vi "UHR-Fleezers Control (fpga) - 9.4.vi"() -> ()   [LabVIEW 2009]
doc: "UHR-Fleezers Instrument Control Code (fpga)"
uses:
  <vilib>/Platform/TimedLoop/XDataNode/XDataNode.xnode
  <vilib>/Platform/TimedLoop/XDataNode/loadlvalarms.vi
  <vilib>/Platform/TimedLoop/XDataNode/timing_clust.ctl
  <vilib>/Platform/TimedLoop/XDataNode/nitl_modes.ctl
  <vilib>/Platform/TimedLoop/XDataNode/wakeup.ctl
  <vilib>/eio/EIONode/EIONode.xnode
  <vilib>/rvi/eio/nirviEIOImplementation/nirviEIOImplementation.xnode
  <vilib>/rvi/eio/common/nirviEmuTemplateMethod_noerrors.vi
  <vilib>/rvi/eio/common/nirviEmuClasses.ctl
  <vilib>/eio/EIOMethodNode/EIOMethodNode.xnode
  <vilib>/rvi/eio/nirviEIOMethodImplementation/nirviEIOMethodImplementation.xnode
  <vilib>/rvi/DataTransferAndStorage/Container/XNode/niFpgaContainer.xnode
  <vilib>/rvi/interface/RandomDataEmulation/niFpgaRandomDataHandleErrors.vi
  <vilib>/rvi/interface/RandomDataEmulation/nirviRandomDataFPGAFIFO.vi
  <vilib>/rvi/DataTransferAndStorage/Container/Common/niFpgaContainerMethod.ctl
  <vilib>/rvi/DataTransferAndStorage/Container/Common/niFpgaTransferTypeControl.ctl
  <vilib>/Platform/TimedLoop/XDataNode/XDNodeRunTimeDep.lvlib
panel:
  in  "Tab Control":T1(tab)=enum."APD Counting"
  in  "AI Averages":u16=1 min=1 step=1
  in  "AI1 Sets to FIFO":T2={"Set 1"=TRUE, "Set 2"=TRUE, "Set 3"=FALSE}
  in  "N of AI1 Int Acq Sets":i16=2 min=1 max=3 step=1
  out "Number of AI channels":i16
  out "AI Late Counter":u32
  in  "ai count":u32=400
  out "AI late?":bool
  in  "+ phase":bool
  in  "Phase count adjustment":i16
  out "Relative phase":i16
  in  "DMA buffer timeout":i32
  in  "AI to FIFO":bool
  in  "Tab Control 2":T3(tab)
  in  "Swap F1 and F2":bool
  in  "Freq or Amp switch first":bool=TRUE
  in  "Cont. Scan":bool
  in  "Abort scan":bool
  in  "Cycles per step":u64
  in  "Scan BD":bool
  in  "Number of scans":u16
  in  "Scan steps":u64
  in  "Scan freq.  increment":i64
  out "Scanning":bool
  in  "Start scan":bool
  in  "OSK Bd 1":bool
  in  "Reset Bd 1":bool
  in  "RD":bool
  in  "PMODE":bool
  in  "OSK Bd 2":bool
  in  "Reset Bd 2":bool
  in  "Direct RF Box \nCommunication":bool
  in  "Data BD 2":u8 format="%08b"
  in  "Data BD 1":u8 format="%08b"
  in  "Address":u8 format="%02x"
  in  "Update Data":bool
  in  "FPGA Controls\n RF Box":bool
  in  "Number Interlace Cycles":u8=2 min=1 max=3
  in  "Interlace Off Parameters":u8=1 min=1 max=3
  in  "Interlace ON/OFF":bool
  out "DIO Relative phase":i16
  in  "Phase count adjustment (DIO)":i16
  in  "+ phase (DIO)":bool
  out "DIO Late Counter":u32
  out "DIO Late?":bool
  in  "DIO count 1 (ticks)":u32=400
  in  "DIO count 2 (ticks)":u32=400
  in  "DIO count 3 (ticks)":u32=400
  out "AI2 Y Sum Set 2":i16
  out "AI2 Y Sum Set 1":i16
  in  "FB Gains Set 1":T4={"proportional gain (Kc)"=10, "integral gain (Kc*Ts/Ti)"=5, "derivative gain (Kc*Td/Ts)"=0}
  in  "FB Setpoint Set 1":i16 min=0 step=1
  in  "FB Reset Set 1":bool
  in  "FB On/Off Set 1":bool
  in  "FB Reset Set 2":bool
  in  "FB On/Off Set 2":bool
  in  "FB Setpoint Set 2":i16 min=0 step=1
  in  "FB Gains Set 2":T4={"proportional gain (Kc)"=10, "integral gain (Kc*Ts/Ti)"=5, "derivative gain (Kc*Td/Ts)"=0}
  in  "FB output range 2":cluster{"output high":i16, "output low":i16}={"output high"=3000, "output low"=0}
  in  "FB output range 1":cluster{"output high":i16, "output low":i16}={"output high"=3000, "output low"=0}
  out "Scan I":u64
  in  "Amp switch delay":u16=5
  in  "Freq switch delay":u16
  in  "BD 2 Amplitude 1":u16
  in  "BD 1 Amplitude 1":u16
  in  "BD 2 Frequency 1":u64
  in  "BD 1 Frequency 1":u64
  in  "BD 2 Amplitude 2":u16
  in  "BD 1 Amplitude 2":u16
  in  "BD 2 Frequency 2":u64
  in  "BD 1 Frequency 2":u64
  in  "BD 2 Amplitude 3":u16
  in  "BD 1 Amplitude 3":u16
  in  "BD 2 Frequency 3":u64
  in  "BD 1 Frequency 3":u64
  out "Numeric":i32
  out "AO2 2":i16
  out "AO1 2":i16
  in  "1D or 2D Scan?":bool
  in  "Abort scan (MCL)":bool
  in  "MCL Scan Axis":bool
  in  "Cont. Scan (MCL)":bool
  out "Scan I (MCL)":u64
  in  "Number of scans (MCL)":u16
  out "Scanning MCL":bool
  in  "Scan steps (MCL)":u64
  in  "Cycles per step (MCL)":u64
  in  "Scan freq.  increment (MCL)":i16
  in  "Start scan (MCL)":bool
  in  "AO2":i16
  in  "AO1":i16
  out "MCL Late Counter":u32
  out "MCL Late?":bool
  in  "MCL count":u32=800
  out "MCL Relative Phase":i16
  in  "Phase count adjustment (MCL)":i16
  in  "+ phase (MCL)":bool
  in  "APD2 Trigger on Edge?":bool=TRUE
  in  "APD1 Trigger on Edge?":bool=TRUE
  in  "APD Gate Operating Mode":u8 max=2 step=1
  in  "Invert APD Gate":bool
  in  "APD Gate OFF Count":u32=100
  in  "APD Gate ON Count":u32=300
  out "APD 1 Gate Late Counter":u32
  out "APD 1 Gate Late?":bool
  out "APD 1 Gate Relative Phase":i16
  in  "Phase count adjustment (APD 1 Gate)":i16
  in  "+ phase (APD 1 Gate)":bool
  out "APD 2 Counts 0":u32
  out "APD 2 Counts 1":u32
  out "APD 1 Counts 0":u32
  out "APD 1 Counts 1":u32
  out "APD out state":bool
  in  "APD 2 AO offset":i16
  in  "APD 1 AO offset":i16
  in  "APD 2 AO scale factor":i16=1
  in  "APD 1 AO scale factor":i16=1
  in  "APD to FIFO":bool
  in  "APD Acq Rate Count":u32=20000000
  out "APD Acq Late Counter":u32
  out "APD Acq Late?":bool
  out "APD Acq Relative Phase":i16
  in  "Phase Count Adjustment (APD Acq)":i16
  in  "+ phase (APD Acq)":bool
  in  "Phase count adjustment (APD 2 Gate)":i16
  out "APD 2 Gate Late Counter":u32
  out "APD 2 Gate Late?":bool
  out "APD 2 Gate Relative Phase":i16
  in  "+ phase (APD 2 Gate)":bool
  in  "Green Filter Flipper":bool
  out "Green FB Signals":T5
  in  "Green FB Count":u32=1200
  out "Green Late Counter":u32
  out "Green FB Late?":bool
  out "Green FB Relative Phase":i16
  in  "Phase count adjustment (Green FB)":i16=10
  in  "+ phase (Green FB)":bool
  out "Green FB Sum":i16
  in  "Green int current ON count adj":u32=150
  in  "Current Out":u16=30000
  in  "Green FB On/Off":bool
  in  "Green FB Setpoint":i16=250 min=0 step=1
  in  "Green FB Gains":T4={"proportional gain (Kc)"=10, "integral gain (Kc*Ts/Ti)"=5, "derivative gain (Kc*Td/Ts)"=0}
  in  "Green FB Reset":bool
  in  "Operating Mode 2":u8=2 max=2 step=1
  in  "Invert GI 2":bool
  in  "Green interlace OFF count 2":u32=900
  in  "Green interlace ON count 2":u32=300
  out "GI Late Counter 2":u32
  out "GI Late? 2":bool
  out "GI Relative phase 2":i16
  in  "Phase count adjustment (GI) 2":i16=20
  in  "+ phase (GI) 2":bool
  in  "Green interlace OFF count":u32=100
  out "GI Relative phase":i16
  in  "Phase count adjustment (GI)":i16
  in  "+ phase (GI)":bool
  out "GI Late?":bool
  in  "Green interlace ON count":u32=300
  out "GI Late Counter":u32
  in  "Invert GI":bool
  in  "Operating Mode":u8 max=2 step=1
  in  "Connector0/DIO9":bool
  in  "Connector1/DIO32":bool
  in  "Connector1/DIO33":bool
  in  "Connector1/DIO34":bool
  in  "Chassis2/Mod4/AO1":u16
  in  "Extra DO Counts":u32=40000
  # "Only one of these can be on\nat a time:"
  # "Raster Scan AOD"
  # "1 (X)"
  # "2 (Y)"
  # "IR Intensity Feedback (RF BD 1)"
  # "AO1 (Y)"
  # "2D"
  # "1D"
  # "AO2 (X)"
  # "APD AO for aligning"
  # "Detection Loop"
  # "Green fluorescent laser digital gate interlacing loop"
  # "0 Forced ON\n1 Forced OFF\n2 Interlacing"
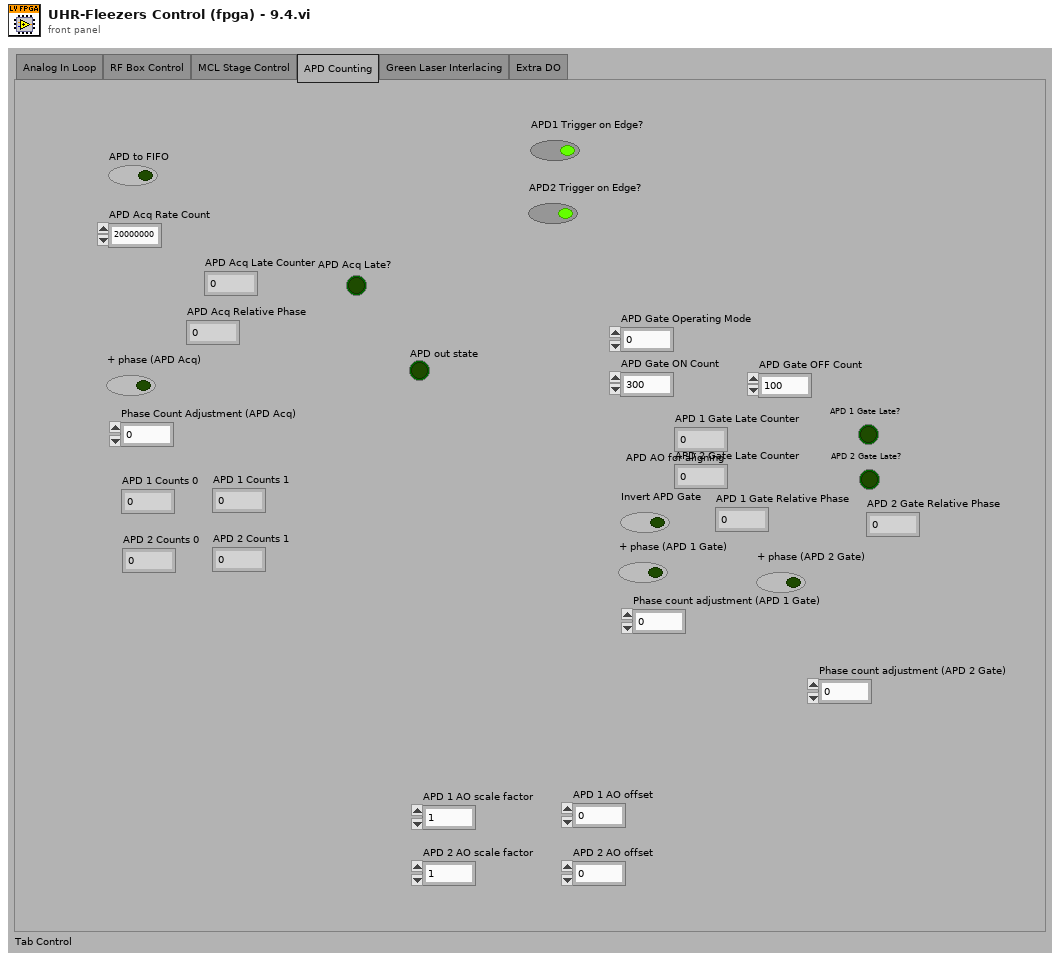
[diagram p1: front panel]
types:
  T1 = enum32{"Analog In Loop", "RF Box Control", "MCL Stage Control", "APD Counting", "Green Laser Interlacing", "Extra DO"}
  T2 = cluster{"Set 1":bool, "Set 2":bool, "Set 3":bool}
  T3 = enum32{"Controls", "Interlacing Frequency and Amplitude Values"}
  T4 = cluster{"proportional gain (Kc)":i16, "integral gain (Kc*Ts/Ti)":i16, "derivative gain (Kc*Td/Ts)":i16}
  T5 = cluster{"Green FB Ch 0":i16, "Green FB Ch 1":i16, "Green FB Ch 2":i16}
  T6 = typedef "nirviEmuClasses.ctl" = enum16{"IO Read", "IO Write", "Method", "Property Read", "Property Write"}
  T7 = typedef "XDNodeRunTimeDep.lvlib/timing_clust.ctl" = cluster{"Expected End [f-1]":u64, "Actual End [f-1]":u64, "Finished Late? [f-1]":bool, "Expected End [i-1]":u64, "Actual End [i-1]":u64, "Finished Late? [i-1]":bool, "Expected Start [i]":u64, "Actual Start [i]":u64, "Expected Start [f]":u64, "Actual Start [f]":u64, "Source Name":string, "Structure Name":string, "Period":i64, "Deadline":i64, "Offset":i64, "Start":i64, "Priority":i32, "Timeout":i32, "Mode":T8, "Wakeup Reason":T9, "Error":errorcluster, "Source Type":string, "Secondary Source Type":string, "Global End Time":u64, "Global Start Time":u64, "Frame Duration":u64, "Iteration Duration":u64, "Assigned CPU":i32, "I/O Scan Engine Mode":u32}
  T8 = typedef "XDNodeRunTimeDep.lvlib/nitl_modes.ctl" = enum32{"No Change", "Process missed periods, maintain original phase", "Discard missed periods, maintain original phase", "Process missed periods, ignore original phase", "Discard missed periods, ignore original phase"}
  T9 = typedef "XDNodeRunTimeDep.lvlib/wakeup.ctl" = enum32{"Normal", "Aborted", "Asynchronous wakeup", "Timing source error", "Timed loop error", "Timeout"}
  T10 = typedef "niFpgaContainerMethod.ctl" = enum16{"Write", "Read", "Clear", "Get Number of Elements to Write", "Get Number of Elements to Read", "Enable", "Disable", "Flush and Disable", "Get Stream State"}
  T11 = typedef "niFpgaTransferTypeControl.ctl" = enum16{"Target-Scoped", "Host to Target - DMA", "Target to Host - DMA", "Peer to Peer Reader", "Peer to Peer Writer", "Bidirectional"}
  T12 = cluster{"Chassis2/Mod1/AI0":i16, "Chassis2/Mod1/AI1":i16, "Chassis2/Mod1/AI2":i16}
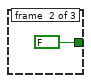
[diagram p2: hidden frame]
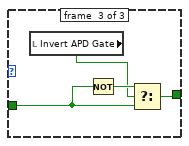
[diagram p3: hidden frame]
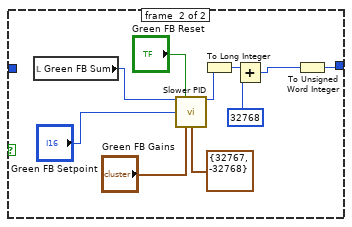
[diagram p4: hidden frame]
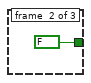
[diagram p5: hidden frame]
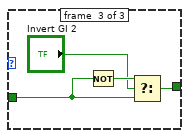
[diagram p6: hidden frame]
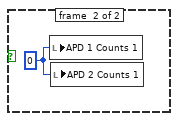
[diagram p7: hidden frame]
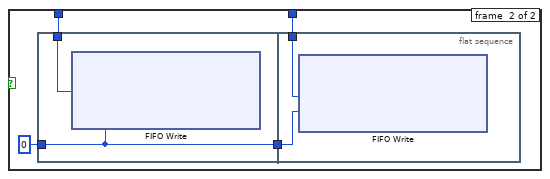
[diagram p8: hidden frame]
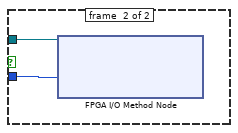
[diagram p9: hidden frame]
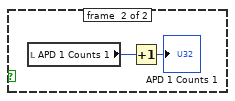
[diagram p10: hidden frame]
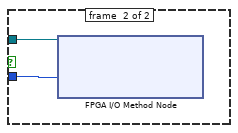
[diagram p11: hidden frame]
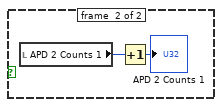
[diagram p12: hidden frame]
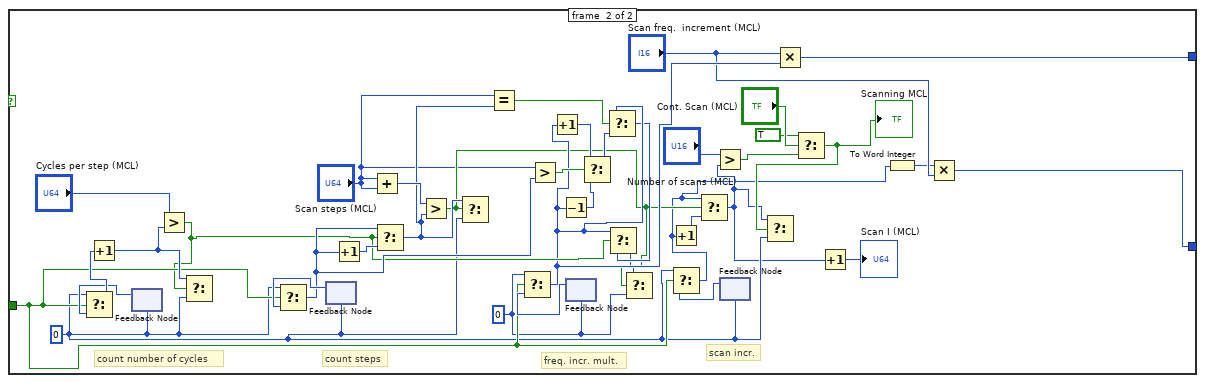
[diagram p13: hidden frame]
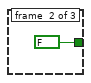
[diagram p14: hidden frame]
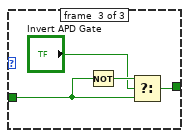
[diagram p15: hidden frame]
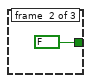
[diagram p16: hidden frame]
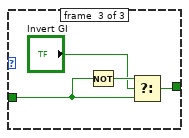
[diagram p17: hidden frame]
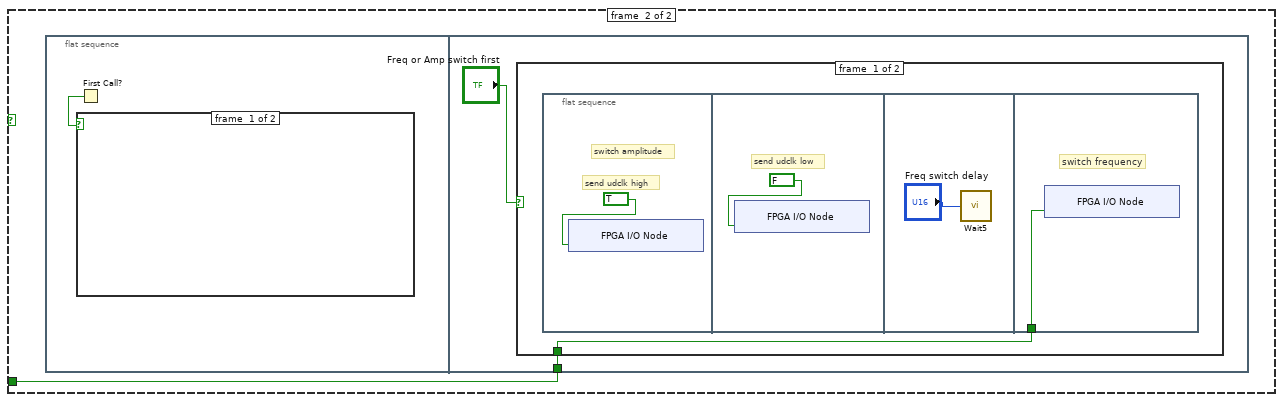
[diagram p18: hidden frame]
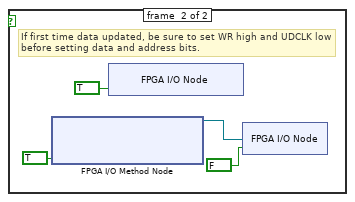
[diagram p19: hidden frame]
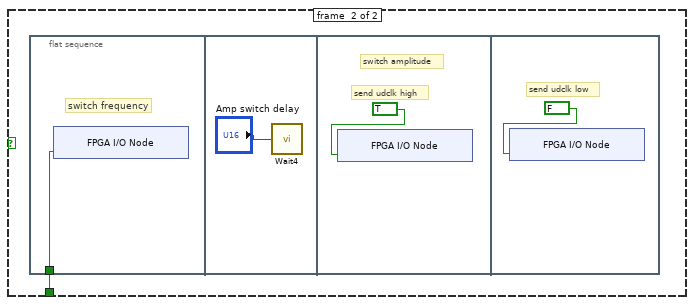
[diagram p20: hidden frame]
diagram:
  w2 = FALSE
  # "timing array current index"
  # "timing array"
  # "timing counter (phase adjusted here)"
  # "late counter"
  n1 = flat-sequence "FPGA initialization to do before running any of the loops" {
    tunnel: [u32 0 ("DIO count 3 (ticks)")] -> w1
    tunnel: [w10] -> _
    frame #0 {
      # "This is a kludge to let host programs know how many channels of data are in the DMA stream.  Set by hand."
      # "Start up expansion chassis early\nto avoid delays later"
      # "This pin controls udclk on the RF boards.\nWhen initially configuring the boards, this pin needs to be\nconfigured as a high impedance input.  Later it will be switched\nto an output."
      # "Initial setting of DIO data and \naddress to low (before reset).  \nThis needs to happen before the other\ncontrol method loops execute."
      n2 = xnode "FPGA I/O Node"("Chassis2/Mod4/AO0"=u16 0) -> ("Chassis2/Mod1/AI0"=w10:i16)  [unwired: 2 in, 2 out]
      n3 = xnode "FPGA I/O Method Node"("Enable"=FALSE) -> ()  [unwired: 1 in, 1 out]
      n4 = xnode "FPGA I/O Node"("Connector1/DIO0"=FALSE, "Connector1/DIO1"=FALSE, "Connector1/DIO2"=FALSE, "Connector1/DIO3"=FALSE, "Connector1/DIO4"=FALSE, "Connector1/DIO5"=FALSE, "Connector1/DIO6"=FALSE, "Connector1/DIO7"=FALSE, "Connector1/DIO8"=FALSE, "Connector1/DIO9"=FALSE, "Connector1/DIO10"=FALSE, "Connector1/DIO11"=FALSE, "Connector1/DIO12"=FALSE, "Connector1/DIO13"=FALSE, "Connector1/DIO15"=FALSE, "Connector1/DIO20"=FALSE, "Connector1/DIO21"=FALSE, "Connector1/DIO22"=FALSE, "Connector1/DIO23"=FALSE, "Connector1/DIO24"=FALSE, "Connector1/DIO25"=FALSE, "Connector1/DIO26"=FALSE, "Connector1/DIO27"=FALSE, "Connector1/DIO14"=FALSE) -> ()  [unwired: 24 in, 24 out]
      "Number of AI channels" <- i16 12 ("Number of AI channels")
    }
  }
  n5 = local read "AO1"() -> (w6:i16)
  n6 = local read "AO2"() -> (w5:i16)
  n7 = node-c288() -> (w4:T7)  [unwired: 1 in]
  n8 = while "APD 1 Counter" {
    tunnel: w1 -> [_]
    stop <- FALSE stop-if-true
    n9 = flat-sequence {
      frame #0 {
        n10 = case shown="False" "APD1 Trigger on Edge?" {
          tunnel: refnum<k21> "Connector0/DIO0" ("APD 1 DO") -> [w398 w423]
          tunnel: -1 ("Timeout") -> [w397 w422]
          frame #0 {
            n11 = xnode "FPGA I/O Method Node"("FPGA I/O In"=w398, "Timeout"=w397) -> ()  [unwired: 2 out]
          }
          frame #1 {
            n12 = xnode "FPGA I/O Method Node"("FPGA I/O In"=w423, "Timeout"=w422) -> ()  [unwired: 2 out]
          }
        }
      }
      frame #1 {
        n13 = local read "APD out state"() -> (w447:bool)
        n14 = case shown="False" w447 {
          frame #0 {
            n15 = local read "APD 1 Counts 0"() -> (w449:u32)
            n16 = Increment(x=w449) -> (x+1=→"APD 1 Counts 0":u32)
          }
          frame #1 {
            n17 = local read "APD 1 Counts 1"() -> (w451:u32)
            n18 = Increment(x=w451) -> (x+1=→"APD 1 Counts 1":u32)
          }
        }
      }
    }
  }
  n19 = while "APD 2 Counter" {
    tunnel: w1 -> [_]
    stop <- FALSE stop-if-true
    n20 = flat-sequence {
      frame #0 {
        n21 = case shown="False" "APD2 Trigger on Edge?" {
          tunnel: refnum<k21> "Connector0/DIO1" ("APD 2 DO") -> [w457 w482]
          tunnel: -1 ("Timeout") -> [w456 w481]
          frame #0 {
            n22 = xnode "FPGA I/O Method Node"("FPGA I/O In"=w457, "Timeout"=w456) -> ()  [unwired: 2 out]
          }
          frame #1 {
            n23 = xnode "FPGA I/O Method Node"("FPGA I/O In"=w482, "Timeout"=w481) -> ()  [unwired: 2 out]
          }
        }
      }
      frame #1 {
        n24 = local read "APD out state"() -> (w506:bool)
        n25 = case shown="False" w506 {
          frame #0 {
            n26 = local read "APD 2 Counts 0"() -> (w508:u32)
            n27 = Increment(x=w508) -> (x+1=→"APD 2 Counts 0":u32)
          }
          frame #1 {
            n28 = local read "APD 2 Counts 1"() -> (w510:u32)
            n29 = Increment(x=w510) -> (x+1=→"APD 2 Counts 1":u32)
          }
        }
      }
    }
  }
  n30 = while "APD 2 Gating" {
    shift-right: [w514] -> _
    shift-left: w1 -> [w519]
    shift-right: [w513] -> _
    shift-left: w2 -> [w511]
    stop <- FALSE stop-if-true
    n31 = flat-sequence {
      tunnel: w519 -> [w522]
      tunnel: [w523] -> w517
      tunnel: [w522] -> w515
      tunnel: [w521] -> w512
      tunnel: w511 -> [w521]
      tunnel: [w526] -> w518
      tunnel: w517 -> [w526]
      tunnel: [w525] -> w516
      tunnel: w515 -> [w525]
      tunnel: w512 -> [w524]
      tunnel: [w580] -> w514
      tunnel: w518 -> [w598]
      tunnel: w516 -> [w596]
      tunnel: [w585] -> w513
      frame #0 {
        n32 = call "Loop Timer8"("Count(Ticks)"=w522) -> ("Tick Count(Ticks)"=w523:u32)
      }
      frame #1 {
        # "(need 4 channels/APD)"
        n33 = xnode "FPGA I/O Node"("Connector0/DIO8"=w524, "Connector0/DIO9"=w524, "Connector0/DIO10"=w524, "Connector0/DIO11"=w524) -> ()  [unwired: 4 in, 4 out]
      }
      frame #2 {
        n34 = local read "APD Gate ON Count"() -> (w573:u32)
        n35 = local read "APD Gate OFF Count"() -> (w572:u32)
        n36 = feedback #1(TRUE) -> (w587:bool)
        n37 = feedback #2(w598) -> (w574:u32)
        n38 = Not(x=w587) -> (.not. x?=w584:bool)
        n39 = Subtract(x=w598, y=w574) -> (x-y=w597:u32)
        n40 = Select(t=w573, s=w584, f=w572) -> (s? t:f=w589:u32)
        n41 = Subtract(x=w597, y=w596) -> (x-y=w590:u32)
        n42 = Subtract(x=w589, y=w590) -> (x-y=w579:u32)
        n43 = Greater?(x=w590, y=u32 0) -> (0:w592:bool)
        "APD 2 Gate Late?" <- w592
        n44 = Boolean To (0,1)(Boolean="+ phase (APD 2 Gate)") -> (0, 1=w577:i16)
        n45 = Multiply(x=w577, y="Phase count adjustment (APD 2 Gate)") -> (x*y=w575:i16)
        n46 = feedback #3(u32 0) -> (w594:u32)
        n47 = Increment(x=w594) -> (x+1=w593:u32)
        n48 = Select(t=w593, s=w592, f=w594) -> (s? t:f=w591:u32)
        "APD 2 Gate Late Counter" <- w591
        n49 = Add(x=w579, y=w575) -> (x+y=w580:u32)
        n50 = feedback #4(i16 0) -> (w582:i16)
        n51 = Subtract(x=w582, y=w575) -> (x-y=w581:i16)
        "APD 2 Gate Relative Phase" <- w581
        n52 = local read "APD Gate Operating Mode"() -> (w571:u8)
        n53 = case shown="2" w571 {
          tunnel: [TRUE FALSE w604] -> w585
          tunnel: w587 -> [_ _ w602]
          frame #0 {
          }
          frame #1 {
          }
          frame #2 {
            n54 = local read "Invert APD Gate"() -> (w601:bool)
            n55 = Not(x=w602) -> (.not. x?=w603:bool)
            n56 = Select(t=w603, s=w601, f=w602) -> (s? t:f=w604:bool)
          }
        }
      }
    }
  }
  n57 = while "DAQ AI set 1" {
    shift-right: [w605] -> _
    shift-left: w1 -> [w610]
    stop <- FALSE stop-if-true
    n58 = flat-sequence {
      tunnel: w610 -> [w620]
      tunnel: [w621] -> w608
      tunnel: [w620] -> w607
      tunnel: [w631] -> w618
      tunnel: [w630] -> w617
      tunnel: [w629] -> w616
      tunnel: [w628] -> w615
      tunnel: [w627] -> w614
      tunnel: [w626] -> w613
      tunnel: [w625] -> w612
      tunnel: [w624] -> w611
      tunnel: [w623] -> w609
      tunnel: w608 -> [w623]
      tunnel: w607 -> [w622]
      tunnel: [w622] -> w606
      tunnel: [w808] -> w605
      tunnel: w618 -> [w846]
      tunnel: w617 -> [w845]
      tunnel: w616 -> [w829]
      tunnel: w615 -> [w844]
      tunnel: w614 -> [w833]
      tunnel: w613 -> [w832]
      tunnel: w612 -> [w831]
      tunnel: w611 -> [w830]
      tunnel: w609 -> [w825]
      tunnel: w606 -> [w822]
      frame #0 {
        n59 = call "Loop Timer3"("Count(Ticks)"=w620) -> ("Tick Count(Ticks)"=w621:u32)
      }
      frame #1 {
        n60 = xnode "FPGA I/O Node"("Connector1/DIO31"=TRUE ("Connector1/DIO33")) -> ("Connector0/AI0"=w631:i16, "Connector0/AI1"=w630:i16, "Connector0/AI2"=w629:i16, "Connector0/AI3"=w628:i16, "Connector0/AI4"=w627:i16, "Connector0/AI5"=w626:i16, "Connector0/AI6"=w625:i16, "Connector0/AI7"=w624:i16)  [unwired: 9 in, 9 out]
      }
      frame #2 {
        # "Adjust phase after data acquired if button pressed"
        n61 = feedback #5(i16 1) -> (w837:i16)
        n62 = Increment(x=w837) -> (x+1=w843:i16)
        n63 = Greater?(x=w843, y="N of AI1 Int Acq Sets") -> (0:w840:bool)
        n64 = Select(t=i16 1, s=w840, f=w843) -> (s? t:f=w842:i16)
        n65 = feedback #6(FALSE ("AI to FIFO")) -> (w827:bool)
        n66 = case shown="1, Default" w837 {
          tunnel: w829 -> [w849 w853 _]
          tunnel: "AI1 Sets to FIFO" -> [w851 w855 w858]
          tunnel: [w850 w854 w857] -> w834
          tunnel: ["AI to FIFO" w852 w856] -> w826
          tunnel: w827 -> [_ w852 w856]
          frame #0 {
            n67 = Unbundle By Name(w851) -> ("Set 1"=w850:bool)
            "AI2 Y Sum Set 1" <- w849
          }
          frame #1 {
            n68 = Unbundle By Name(w855) -> ("Set 2"=w854:bool)
            "AI2 Y Sum Set 2" <- w853
          }
          frame #2 {
            n69 = Unbundle By Name(w858) -> ("Set 3"=w857:bool)
          }
        }
        n70 = And(x=w834, y=w826) -> (x .and. y?=w836:bool)
        n71 = case shown="True" w836 {
          tunnel: w846 -> [_ w863]
          tunnel: w845 -> [_ w864]
          tunnel: w829 -> [_ w865]
          tunnel: w844 -> [_ w866]
          tunnel: w833 -> [_ w870]
          tunnel: w832 -> [_ w869]
          tunnel: w831 -> [_ w868]
          tunnel: w830 -> [_ w867]
          frame #0 {
          }
          frame #1 {
            n72 = Greater?(x="AI Averages", y=u16 1) -> (0:w861:bool)
            n73 = case shown="True" w861 {
              tunnel: w870 -> [w881 w938]
              tunnel: w869 -> [w880 w937]
              tunnel: w868 -> [w879 w936]
              tunnel: w867 -> [w878 w935]
              tunnel: w866 -> [w877 w934]
              tunnel: w865 -> [w882 w933]
              tunnel: w864 -> [w883 w932]
              tunnel: w863 -> [w884 w931]
              tunnel: "AI Averages" -> [_ w918]
              tunnel: "DMA buffer timeout" -> [w872 w915]
              frame #0 {
                n74 = Join Numbers(hi=w884, lo=w883) -> ((hi.lo)=w876:u32)
                n75 = Join Numbers(hi=w882, lo=w877) -> ((hi.lo)=w875:u32)
                n76 = Join Numbers(hi=w881, lo=w880) -> ((hi.lo)=w874:u32)
                n77 = Join Numbers(hi=w879, lo=w878) -> ((hi.lo)=w873:u32)
                n78 = Build Array(w876, w875, w874, w873) -> (w871:u32[])
                n79 = for {
                  tunnel: w871 -> [w886] mode=indexing
                  tunnel: w872 -> [w887]
                  n80 = To Unsigned Long Integer(number=w886) -> (unsigned 32bit integer=w885:u32)
                  n81 = xnode ("FIFO Write")("Element"=w885, "Timeout"=w887) -> ()  [unwired: 1 in, 2 out]
                }
              }
              frame #1 {
                w922 = u16 0
                n82 = To Long Integer(number=w931) -> (32bit integer=w924:i32)
                n83 = To Long Integer(number=w932) -> (32bit integer=w941:i32)
                n84 = To Long Integer(number=w933) -> (32bit integer=w940:i32)
                n85 = To Long Integer(number=w934) -> (32bit integer=w939:i32)
                n86 = To Long Integer(number=w938) -> (32bit integer=w930:i32)
                n87 = To Long Integer(number=w937) -> (32bit integer=w929:i32)
                n88 = To Long Integer(number=w936) -> (32bit integer=w928:i32)
                n89 = To Long Integer(number=w935) -> (32bit integer=w927:i32)
                n90 = Build Array(w924, w941, w940, w939, w930, w929, w928, w927) -> (w913:i32[])
                n91 = feedback #7(w913) -> (w926:i32[])
                n92 = Add(x=w913, y=w926) -> (x+y=w925:i32[])
                n93 = feedback #8(w922) -> (w920:u16)
                n94 = Increment(x=w920) -> (x+1=w917:u16)
                n95 = Equal?(x=w917, y=u16 1) -> (x = y?=w916:bool)
                n96 = Select(t=w913, s=w916, f=w925) -> (s? t:f=w914:i32[])
                n97 = Greater Or Equal?(x=w917, y=w918) -> (x >= y?=w919:bool)
                n98 = Select(t=w922, s=w919, f=w917) -> (s? t:f=w921:u16)
                n99 = case shown="True" w919 {
                  tunnel: w914 -> [_ w943]
                  tunnel: w915 -> [_ w942]
                  frame #0 {
                  }
                  frame #1 {
                    n100 = for {
                      tunnel: w943 -> [w945] mode=indexing
                      tunnel: w942 -> [w946]
                      n101 = To Unsigned Long Integer(number=w945) -> (unsigned 32bit integer=w944:u32)
                      n102 = xnode ("FIFO Write")("Element"=w944, "Timeout"=w946) -> ()  [unwired: 1 in, 2 out]
                    }
                  }
                }
              }
            }
          }
        }
        n103 = feedback #9(w825) -> (w824:u32)
        n104 = Subtract(x=w825, y=w824) -> (x-y=w823:u32)
        n105 = Subtract(x=w823, y=w822) -> (x-y=w819:u32)
        n106 = Subtract(x="ai count", y=w819) -> (x-y=w809:u32)
        n107 = Greater?(x=w819, y=u32 0) -> (0:w817:bool)
        "AI late?" <- w817
        n108 = feedback #10(u32 0) -> (w815:u32)
        n109 = Increment(x=w815) -> (x+1=w814:u32)
        n110 = Select(t=w814, s=w817, f=w815) -> (s? t:f=w816:u32)
        "AI Late Counter" <- w816
        n111 = xnode "I/O Node"("Connector1/DIO31"=FALSE ("Connector1/DIO34")) -> ()  [unwired: 1 in, 1 out]
        n112 = Boolean To (0,1)(Boolean="+ phase") -> (0, 1=w811:i16)
        n113 = Multiply(x=w811, y="Phase count adjustment") -> (x*y=w805:i16)
        n114 = feedback #11(i16 0) -> (w807:i16)
        n115 = Add(x=w809, y=w805) -> (x+y=w808:u32)
        n116 = Subtract(x=w807, y=w805) -> (x-y=w806:i16)
        "Relative phase" <- w806
      }
    }
  }
  n117 = while "RF box board DIO control: parallel communication" {
    shift-right: [w991] -> _
    shift-left: w1 -> [w990]
    shift-right: [w989] -> _
    shift-left: FALSE ("Swap F1 and F2") -> [w988]
    stop <- FALSE stop-if-true
    n118 = flat-sequence {
      tunnel: w988 -> [w995]
      tunnel: w990 -> [w993]
      tunnel: [w995] -> w987
      tunnel: [w994] -> w986
      tunnel: [w993] -> w985
      tunnel: [w1001] -> w991
      tunnel: [w1000] -> w989
      tunnel: w987 -> [w999]
      tunnel: w986 -> [w997]
      tunnel: w985 -> [w996]
      frame #0 {
        n119 = call "Loop Timer"("Count(Ticks)"=w993) -> ("Tick Count(Ticks)"=w994:u32)
      }
      frame #1 {
        n120 = flat-sequence {
          tunnel: ["FPGA Controls\n RF Box"] -> w998
          tunnel: w999 -> [w1002]
          tunnel: [w1151] -> w1001
          tunnel: [w1171] -> w1000
          tunnel: w998 -> [w1170]
          tunnel: w997 -> [w1164]
          tunnel: w996 -> [w1161]
          frame #0 {
            n121 = case shown="True" "FPGA Controls\n RF Box" {
              tunnel: w1002 -> [_ w1004]
              frame #0 {
              }
              frame #1 {
                n122 = flat-sequence {
                  tunnel: w1004 -> [w1049]
                  frame #0 {
                    n123 = First Call?() -> (First Call?: T/F=w1005:bool)
                    n124 = case shown="True" w1005 {
                      frame #0 {
                      }
                      frame #1 {
                        # "If first time data updated, be sure to set WR high and UDCLK low\nbefore setting data and address bits."
                        n125 = xnode "FPGA I/O Method Node"("Enable"=TRUE) -> ("FPGA I/O Out"=w1007:refnum<k21>)  [unwired: 1 in]
                        n126 = xnode "FPGA I/O Node"("Connector1/DIO15"=TRUE) -> ()  [unwired: 1 in, 1 out]
                        n127 = xnode "FPGA I/O Node"("I/O Item"=FALSE ("Connector1/DIO30"), "FPGA I/O In"=w1007) -> ()  [unwired: 1 out]
                      }
                    }
                  }
                  frame #1 {
                    n128 = case shown="True" "Freq or Amp switch first" {
                      tunnel: w1049 -> [w1051 w1095]
                      frame #0 {
                        n129 = flat-sequence {
                          tunnel: w1051 -> [w1081]
                          frame #0 {
                            # "switch amplitude"
                            # "send udclk high"
                            n130 = xnode "FPGA I/O Node"("Connector1/DIO30"=TRUE ("Connector1/DIO15")) -> ()  [unwired: 1 in, 1 out]
                          }
                          frame #1 {
                            # "send udclk low"
                            n131 = xnode "FPGA I/O Node"("Connector1/DIO30"=FALSE ("Connector1/DIO15")) -> ()  [unwired: 1 in, 1 out]
                          }
                          frame #2 {
                            n132 = call "Wait5"("Count(Ticks)"="Freq switch delay") -> ()  [unwired: 1 out]
                          }
                          frame #3 {
                            # "switch frequency"
                            n133 = xnode "FPGA I/O Node"("Connector1/DIO36"=w1081) -> ()  [unwired: 1 in, 1 out]
                          }
                        }
                      }
                      frame #1 {
                        n134 = flat-sequence {
                          tunnel: w1095 -> [w1096]
                          frame #0 {
                            # "switch frequency"
                            n135 = xnode "FPGA I/O Node"("Connector1/DIO36"=w1096) -> ()  [unwired: 1 in, 1 out]
                          }
                          frame #1 {
                            n136 = call "Wait4"("Count(Ticks)"="Amp switch delay") -> ()  [unwired: 1 out]
                          }
                          frame #2 {
                            # "switch amplitude"
                            # "send udclk high"
                            n137 = xnode "FPGA I/O Node"("Connector1/DIO30"=TRUE ("Connector1/DIO15")) -> ()  [unwired: 1 in, 1 out]
                          }
                          frame #3 {
                            # "send udclk low"
                            n138 = xnode "FPGA I/O Node"("Connector1/DIO30"=FALSE ("Connector1/DIO15")) -> ()  [unwired: 1 in, 1 out]
                          }
                        }
                      }
                    }
                  }
                }
              }
            }
          }
          frame #1 {
            # "This is the prior cycle's on time"
            # "increment timing\nindex, reset to 0 if \nend of matrix"
            # "Reset to begginning (1) when number of cycles reached."
            # "timing index"
            # "build byte stacks for writing data\n(must correspond to addresses array constant)"
            # "Timing housekeeping"
            # "Adjust phase if late\n(maintains constant phase relationship between cycles)"
            n139 = feedback #12(u8 0 ("t")) -> (w1167:u8)
            n140 = Increment(x=w1167) -> (x+1=w1211:u8)
            n141 = Increment(x="Number Interlace Cycles") -> (x+1=w1206:u8)
            n142 = Equal?(x=w1211, y=w1206) -> (x = y?=w1213:bool)
            n143 = Select(t=u8 1, s=w1213, f=w1211) -> (s? t:f=w1166:u8)
            n144 = Increment(x=w1166) -> (x+1=w1208:u8)
            n145 = Equal?(x=w1208, y=w1206) -> (x = y?=w1209:bool)
            n146 = Select(t=u8 1, s=w1209, f=w1208) -> (s? t:f=w1205:u8)
            n147 = Select(t=w1205, s="Interlace ON/OFF", f="Interlace Off Parameters") -> (s? t:f=w1189:u8)
            n148 = case shown="1, Default" w1189 {
              tunnel: [w1285 "BD 1 Frequency 2" "BD 1 Frequency 3"] -> w1201
              tunnel: [w1284 "BD 2 Frequency 2" "BD 2 Frequency 3"] -> w1190
              tunnel: ["BD 2 Amplitude 1" "BD 2 Amplitude 2" "BD 2 Amplitude 3"] -> w1139
              tunnel: [w1273 w1343 "BD 1 Amplitude 3"] -> w1142
              frame #0 {
                w1280 = u8 0 ("f")
                n149 = local read "Scanning"() -> (w1286:bool)
                n150 = Or(x=w1286, y="Start scan") -> (x .or. y?=w1278:bool)
                n151 = Not(x="Abort scan") -> (.not. x?=w1276:bool)
                n152 = And(x=w1276, y=w1278) -> (x .and. y?=w1275:bool)
                n153 = case "Raster scan" shown="True" w1275 {
                  tunnel: [i16 0 w1332] -> w1281
                  tunnel: "Start scan" -> [_ w1317]
                  frame #0 {
                    n154 = local write "Scanning"(FALSE ("scanning")) -> ()
                  }
                  frame #1 {
                    w1301 = i64 0
                    w1300 = u64 0
                    # "scan incr."
                    # "freq. incr. mult."
                    # "count steps"
                    # "count number of cycles"
                    n155 = feedback #13(w1300) -> (w1329:u64)
                    n156 = Select(t=w1300, s=w1317, f=w1329) -> (s? t:f=w1331:u64)
                    n157 = Increment(x=w1331) -> (x+1=w1328:u64)
                    n158 = Greater?(x="Cycles per step", y=w1328) -> (0:w1310:bool)
                    n159 = Select(t=w1328, s=w1310, f=w1300) -> (s? t:f=w1327:u64)
                    n160 = feedback #14(w1300) -> (w1326:u64)
                    n161 = Select(t=w1300, s=w1317, f=w1326) -> (s? t:f=w1321:u64)
                    n162 = Increment(x=w1321) -> (x+1=w1325:u64)
                    n163 = Add(x="Scan steps", y="Scan steps") -> (x+y=w1324:u64)
                    n164 = Select(t=w1321, s=w1310, f=w1325) -> (s? t:f=w1305:u64)
                    n165 = Greater?(x=w1324, y=w1305) -> (0:w1304:bool)
                    n166 = Select(t=w1305, s=w1304, f=w1300) -> (s? t:f=w1322:u64)
                    n167 = Equal?(x="Scan steps", y=w1305) -> (x = y?=w1309:bool)
                    n168 = Greater?(x="Scan steps", y=w1321) -> (0:w1320:bool)
                    n169 = feedback #15(w1301) -> (w1323:i64)
                    n170 = Select(t=w1301, s=w1317, f=w1323) -> (s? t:f=w1307:i64)
                    n171 = Increment(x=w1307) -> (x+1=w1319:i64)
                    n172 = Decrement(x=w1307) -> (x-1=w1318:i64)
                    n173 = Select(t=w1319, s=w1320, f=w1318) -> (s? t:f=w1308:i64)
                    n174 = Select(t=w1307, s=w1309, f=w1308) -> (s? t:f=w1306:i64)
                    n175 = Select(t=w1307, s=w1310, f=w1306) -> (s? t:f=w1302:i64)
                    n176 = Select(t=w1302, s=w1304, f=w1301) -> (s? t:f=w1303:i64)
                    n177 = feedback #16(w1300) -> (w1316:u64)
                    n178 = Select(t=w1300, s=w1317, f=w1316) -> (s? t:f=w1312:u64)
                    n179 = Increment(x=w1312) -> (x+1=w1313:u64)
                    n180 = Select(t=w1312, s=w1304, f=w1313) -> (s? t:f=w1311:u64)
                    n181 = Greater?(x="Number of scans", y=w1311) -> (0:w1297:bool)
                    n182 = Multiply(x="Scan freq.  increment", y=w1307) -> (x*y=w1332:i64)
                    n183 = Select(t=TRUE, s="Cont. Scan", f=w1297) -> (s? t:f=w1296:bool)
                    "Scanning" <- w1296
                    n184 = Select(t=w1311, s=w1296, f=w1300) -> (s? t:f=w1314:u64)
                    n185 = Increment(x=w1311) -> (x+1=→"Scan I":u64)
                  }
                }
                n186 = case shown="True" "FB On/Off Set 1" {
                  tunnel: "BD 1 Amplitude 1" -> [w1334 _]
                  tunnel: [w1334 w1335] -> w1273
                  frame #0 {
                  }
                  frame #1 {
                    n187 = local read "AI2 Y Sum Set 1"() -> (w1337:i16)
                    n188 = call "Slower PID.vi"("process variable"=w1337, "reset?"="FB Reset Set 1", "setpoint"="FB Setpoint Set 1", "PID gains (x 2^8)"="FB Gains Set 1", "output range"="FB output range 1") -> ("output"=w1340:i16)  [unwired: 10 out]
                    n189 = To Unsigned Word Integer(number=w1340) -> (unsigned 16bit integer=w1335:u16)
                  }
                }
                n190 = Select(t=w1280, s="Scan BD", f=w1281) -> (s? t:f=w1279:i64)
                n191 = Select(t=w1281, s="Scan BD", f=w1280) -> (s? t:f=w1282:i64)
                n192 = Add(x=w1279, y="BD 2 Frequency 1") -> (x+y=w1284:u64)
                n193 = Add(x="BD 1 Frequency 1", y=w1282) -> (x+y=w1285:u64)
              }
              frame #1 {
                n194 = case shown="True" "FB On/Off Set 2" {
                  tunnel: [w1348 w1349] -> w1343
                  tunnel: "BD 1 Amplitude 2" -> [w1348 _]
                  frame #0 {
                  }
                  frame #1 {
                    n195 = local read "AI2 Y Sum Set 2"() -> (w1354:i16)
                    n196 = call "Slower PID.vi"("process variable"=w1354, "reset?"="FB Reset Set 2", "setpoint"="FB Setpoint Set 2", "PID gains (x 2^8)"="FB Gains Set 2", "output range"="FB output range 2") -> ("output"=w1351:i16)  [unwired: 10 out]
                    n197 = To Unsigned Word Integer(number=w1351) -> (unsigned 16bit integer=w1349:u16)
                  }
                }
              }
              frame #2 {
              }
            }
            n198 = feedback #17(w1164) -> (w1163:u32)
            n199 = Subtract(x=w1164, y=w1163) -> (x-y=w1162:u32)
            n200 = Select(t=w1166, s="Interlace ON/OFF", f="Interlace Off Parameters") -> (s? t:f=w1204:u8)
            n201 = Subtract "The error"(x=w1162, y=w1161) -> (x-y=w1159:u32)
            n202 = case shown="3" w1204 {
              tunnel: ["DIO count 1 (ticks)" "DIO count 2 (ticks)" "DIO count 3 (ticks)"] -> w1160
              frame #0 {
              }
              frame #1 {
              }
              frame #2 {
              }
            }
            n203 = Greater?(x=w1159, y=u32 0) -> (0:w1154:bool)
            "DIO Late?" <- w1154
            n204 = feedback #18(u32 0) -> (w1156:u32)
            n205 = Increment(x=w1156) -> (x+1=w1155:u32)
            n206 = Select(t=w1155, s=w1154, f=w1156) -> (s? t:f=w1157:u32)
            "DIO Late Counter" <- w1157
            n207 = Subtract(x=w1160, y=w1159) -> (x-y=w1152:u32)
            n208 = Boolean To (0,1)(Boolean="+ phase (DIO)") -> (0, 1=w1149:i16)
            n209 = Multiply(x=w1149, y="Phase count adjustment (DIO)") -> (x*y=w1145:i16)
            n210 = feedback #19(i16 0) -> (w1147:i16)
            n211 = Subtract(x=w1147, y=w1145) -> (x-y=w1146:i16)
            "DIO Relative phase" <- w1146
            n212 = Split Number(x=w1190) -> (hi(x)=w1195:u32, lo(x)=w1194:u32)
            n213 = Split Number(x=w1201) -> (hi(x)=w1200:u32, lo(x)=w1199:u32)
            n214 = Split Number(x=w1195) -> (lo(x)=w1193:u16)  [unwired: 1 out]
            n215 = Split Number(x=w1194) -> (hi(x)=w1192:u16, lo(x)=w1191:u16)
            n216 = Split Number(x=w1200) -> (lo(x)=w1198:u16)  [unwired: 1 out]
            n217 = Split Number(x=w1199) -> (hi(x)=w1197:u16, lo(x)=w1196:u16)
            n218 = Split Number(x=w1142) -> (hi(x)=w1144:u8, lo(x)=w1143:u8)
            n219 = Split Number(x=w1193) -> (hi(x)=w1181:u8, lo(x)=w1180:u8)
            n220 = Split Number(x=w1192) -> (hi(x)=w1179:u8, lo(x)=w1178:u8)
            n221 = Split Number(x=w1191) -> (hi(x)=w1177:u8, lo(x)=w1176:u8)
            n222 = Split Number(x=w1139) -> (hi(x)=w1141:u8, lo(x)=w1140:u8)
            n223 = Add(x=w1152, y=w1145) -> (x+y=w1151:u32)
            n224 = Split Number(x=w1198) -> (hi(x)=w1188:u8, lo(x)=w1187:u8)
            n225 = Split Number(x=w1197) -> (hi(x)=w1186:u8, lo(x)=w1185:u8)
            n226 = Split Number(x=w1196) -> (hi(x)=w1184:u8, lo(x)=w1183:u8)
            n227 = Build Array "BD 1 A Stack"(w1144, w1143) -> (w1173:u8[])
            n228 = Build Array "BD 2 nu Stack"(w1181, w1180, w1179, w1178, w1177, w1176) -> (w1175:u8[])
            n229 = Build Array "BD 2 A Stack"(w1141, w1140) -> (w1172:u8[])
            n230 = Build Array "BD 1 nu Stack"(w1188, w1187, w1186, w1185, w1184, w1183) -> (w1182:u8[])
            n231 = case shown="2" w1189 {
              tunnel: [w1265 w1268] -> w1171
              tunnel: [u8 10 u8 4] -> w1174
              tunnel: "Swap F1 and F2" -> [w1266 w1268]
              frame #0 {
                # "F2"
                n232 = Not(x=w1266) -> (.not. x?=w1265:bool)
              }
              frame #1 {
                # "low chooses F1"
                # "F1"
              }
            }
            n233 = case "If FPGA is controlling (toggling) RF synth" shown="True" w1170 {
              tunnel: w1182 -> [_ w1218]
              tunnel: w1175 -> [_ w1217]
              tunnel: w1174 -> [_ w1216]
              tunnel: w1173 -> [_ w1215]
              tunnel: w1172 -> [_ w1214]
              frame #0 {
              }
              frame #1 {
                # "Write next amp.\n(wait until beginning of next loop iteration to update)"
                n234 = flat-sequence "Update the next F1 and F2 frequency value (the actual frequency won't change until FSK is switched).\nThen load the next amplitude value into buffer, but don't update it until the next cycle." {
                  tunnel: w1218 -> [w1221]
                  tunnel: w1217 -> [w1220]
                  tunnel: w1216 -> [w1219]
                  tunnel: w1215 -> [w1258]
                  tunnel: w1214 -> [w1257]
                  frame #0 {
                    n235 = for {
                      tunnel: w1221 -> [w1227] mode=indexing
                      tunnel: w1220 -> [w1226] mode=indexing
                      tunnel: w1219 -> [w1224]
                      i -> [w1225]
                      # "Write next freq."
                      n236 = To Unsigned Byte Integer(number=w1225) -> (unsigned 8bit integer=w1222:u8)
                      n237 = Add(x=w1224, y=w1222) -> (x+y=w1223:u8)
                      n238 = call "write to RF synth bd.vi"("Address Byte"=w1223, "BD 2 Byte"=w1226, "BD 1 Byte"=w1227) -> ()
                    }
                  }
                  frame #1 {
                    # "send udclk high"
                    n239 = xnode "FPGA I/O Node"("Connector1/DIO30"=TRUE ("Connector1/DIO15")) -> ()  [unwired: 1 in, 1 out]
                  }
                  frame #2 {
                    n240 = xnode "FPGA I/O Node"("Connector1/DIO30"=FALSE ("Connector1/DIO15")) -> ()  [unwired: 1 in, 1 out]
                  }
                  frame #3 {
                    n241 = for {
                      tunnel: w1258 -> [w1264] mode=indexing
                      tunnel: w1257 -> [w1263] mode=indexing
                      tunnel: u8 33 -> [w1261]
                      i -> [w1262]
                      n242 = To Unsigned Byte Integer(number=w1262) -> (unsigned 8bit integer=w1259:u8)
                      n243 = Add(x=w1261, y=w1259) -> (x+y=w1260:u8)
                      n244 = call "write to RF synth bd.vi"("Address Byte"=w1260, "BD 2 Byte"=w1263, "BD 1 Byte"=w1264) -> ()
                    }
                  }
                }
              }
            }
          }
        }
      }
    }
  }
  n245 = while "MCL stage control" {
    shift-right: [w1375] -> _
    shift-left: w1 -> [w1378]
    shift-right: [w1368] -> _
    shift-left: w6 -> [w1365]
    shift-right: [w1367] -> _
    shift-left: w5 -> [w1363]
    i -> [w1362]
    stop <- FALSE stop-if-true
    n246 = flat-sequence {
      tunnel: w1378 -> [w1382]
      tunnel: [w1383] -> w1374
      tunnel: [w1382] -> w1372
      tunnel: [w1381] -> w1366
      tunnel: w1365 -> [w1381]
      tunnel: [w1380] -> w1364
      tunnel: w1363 -> [w1380]
      tunnel: w1374 -> [w1387]
      tunnel: [w1387] -> w1373
      tunnel: w1372 -> [w1386]
      tunnel: [w1386] -> w1371
      tunnel: w1366 -> [w1385]
      tunnel: w1364 -> [w1384]
      tunnel: [w1385] -> w1361
      tunnel: [w1384] -> w1360
      tunnel: w1373 -> [w1421]
      tunnel: w1371 -> [w1420]
      tunnel: [w1421] -> w1377
      tunnel: [w1420] -> w1376
      tunnel: [w1419] -> w1370
      tunnel: [w1418] -> w1369
      tunnel: w1361 -> [w1413]
      tunnel: w1360 -> [w1412]
      tunnel: [w1485] -> w1375
      tunnel: w1377 -> [w1499]
      tunnel: w1376 -> [w1496]
      tunnel: w1370 -> [w1488]
      tunnel: w1369 -> [w1487]
      tunnel: [w1488] -> w1368
      tunnel: [w1487] -> w1367
      frame #0 {
        n247 = call "Loop Timer5"("Count(Ticks)"=w1382) -> ("Tick Count(Ticks)"=w1383:u32)
      }
      frame #1 {
        n248 = xnode "FPGA I/O Node"("Connector0/AO1"=w1385, "Connector0/AO2"=w1384) -> ()  [unwired: 2 in, 2 out]
      }
      frame #2 {
        n249 = local read "Scanning MCL"() -> (w1433:bool)
        n250 = Or(x=w1433, y="Start scan (MCL)") -> (x .or. y?=w1428:bool)
        n251 = Not(x="Abort scan (MCL)") -> (.not. x?=w1426:bool)
        n252 = And(x=w1426, y=w1428) -> (x .and. y?=w1425:bool)
        n253 = case "Raster scan" shown="True" w1425 {
          tunnel: [w1434 w1477] -> w1430
          tunnel: "Start scan (MCL)" -> [_ w1462]
          tunnel: [w1434 w1438] -> w1414
          frame #0 {
            w1434 = i16 0
            n254 = local write "Scanning MCL"(FALSE ("scanning")) -> ()
          }
          frame #1 {
            w1448 = i16 0
            w1447 = u64 0
            # "scan incr."
            # "freq. incr. mult."
            # "count steps"
            # "count number of cycles"
            n255 = feedback #20(w1447) -> (w1474:u64)
            n256 = Select(t=w1447, s=w1462, f=w1474) -> (s? t:f=w1476:u64)
            n257 = Increment(x=w1476) -> (x+1=w1473:u64)
            n258 = Greater?(x="Cycles per step (MCL)", y=w1473) -> (0:w1457:bool)
            n259 = Select(t=w1473, s=w1457, f=w1447) -> (s? t:f=w1472:u64)
            n260 = feedback #21(w1447) -> (w1471:u64)
            n261 = Select(t=w1447, s=w1462, f=w1471) -> (s? t:f=w1466:u64)
            n262 = Increment(x=w1466) -> (x+1=w1470:u64)
            n263 = Add(x="Scan steps (MCL)", y="Scan steps (MCL)") -> (x+y=w1469:u64)
            n264 = Select(t=w1466, s=w1457, f=w1470) -> (s? t:f=w1452:u64)
            n265 = Greater?(x=w1469, y=w1452) -> (0:w1451:bool)
            n266 = Select(t=w1452, s=w1451, f=w1447) -> (s? t:f=w1467:u64)
            n267 = Equal?(x="Scan steps (MCL)", y=w1452) -> (x = y?=w1456:bool)
            n268 = Greater?(x="Scan steps (MCL)", y=w1466) -> (0:w1465:bool)
            n269 = feedback #22(w1448) -> (w1468:i16)
            n270 = Select(t=w1448, s=w1462, f=w1468) -> (s? t:f=w1454:i16)
            n271 = Increment(x=w1454) -> (x+1=w1464:i16)
            n272 = Decrement(x=w1454) -> (x-1=w1463:i16)
            n273 = Select(t=w1464, s=w1465, f=w1463) -> (s? t:f=w1455:i16)
            n274 = Select(t=w1454, s=w1456, f=w1455) -> (s? t:f=w1453:i16)
            n275 = Select(t=w1454, s=w1457, f=w1453) -> (s? t:f=w1449:i16)
            n276 = Select(t=w1449, s=w1451, f=w1448) -> (s? t:f=w1450:i16)
            n277 = feedback #23(w1447) -> (w1461:u64)
            n278 = Select(t=w1447, s=w1462, f=w1461) -> (s? t:f=w1436:u64)
            n279 = Increment(x=w1436) -> (x+1=w1458:u64)
            n280 = Select(t=w1436, s=w1451, f=w1458) -> (s? t:f=w1437:u64)
            n281 = Greater?(x="Number of scans (MCL)", y=w1437) -> (0:w1444:bool)
            n282 = Multiply(x="Scan freq.  increment (MCL)", y=w1454) -> (x*y=w1477:i16)
            n283 = Select(t=TRUE, s="Cont. Scan (MCL)", f=w1444) -> (s? t:f=w1443:bool)
            "Scanning MCL" <- w1443
            n284 = Select(t=w1437, s=w1443, f=w1447) -> (s? t:f=w1459:u64)
            n285 = Increment(x=w1437) -> (x+1=→"Scan I (MCL)":u64)
            n286 = To Word Integer(number=w1436) -> (16bit integer=w1439:i16)
            n287 = Multiply(x=w1439, y="Scan freq.  increment (MCL)") -> (x*y=w1438:i16)
          }
        }
        n288 = Select(t=w1414, s="1D or 2D Scan?", f=i16 0) -> (s? t:f=w1415:i16)
        n289 = Select(t=w1415, s="MCL Scan Axis", f=w1430) -> (s? t:f=w1429:i16)
        n290 = Select(t=w1430, s="MCL Scan Axis", f=w1415) -> (s? t:f=w1431:i16)
        n291 = Add(x=w1429, y="AO2") -> (x+y=w1418:i16)
        n292 = Add(x="AO1", y=w1431) -> (x+y=w1419:i16)
        "AO1 2" <- w1413
        "AO2 2" <- w1412
      }
      frame #3 {
        n293 = feedback #24(w1499) -> (w1498:u32)
        n294 = Boolean To (0,1)(Boolean="+ phase (MCL)") -> (0, 1=w1483:i16)
        n295 = Subtract(x=w1499, y=w1498) -> (x-y=w1497:u32)
        n296 = Multiply(x=w1483, y="Phase count adjustment (MCL)") -> (x*y=w1479:i16)
        n297 = Subtract(x=w1497, y=w1496) -> (x-y=w1494:u32)
        n298 = Subtract(x="MCL count", y=w1494) -> (x-y=w1481:u32)
        n299 = feedback #25(i16 0) -> (w1480:i16)
        n300 = Subtract(x=w1480, y=w1479) -> (x-y=w1478:i16)
        "MCL Relative Phase" <- w1478
        n301 = Greater?(x=w1494, y=u32 0) -> (0:w1493:bool)
        "MCL Late?" <- w1493
        n302 = Add(x=w1481, y=w1479) -> (x+y=w1485:u32)
        n303 = feedback #26(u32 0) -> (w1491:u32)
        n304 = Increment(x=w1491) -> (x+1=w1490:u32)
        n305 = Select(t=w1490, s=w1493, f=w1491) -> (s? t:f=w1492:u32)
        "MCL Late Counter" <- w1492
      }
    }
    "Numeric" <- w1362
  }
  n306 = while "APD 1 Gating" {
    shift-right: [w1504] -> _
    shift-left: w1 -> [w1509]
    shift-right: [w1503] -> _
    shift-left: w2 -> [w1501]
    stop <- FALSE stop-if-true
    n307 = flat-sequence {
      tunnel: w1509 -> [w1512]
      tunnel: [w1513] -> w1507
      tunnel: [w1512] -> w1505
      tunnel: [w1511] -> w1502
      tunnel: w1501 -> [w1511]
      tunnel: [w1516] -> w1508
      tunnel: w1507 -> [w1516]
      tunnel: [w1515] -> w1506
      tunnel: w1505 -> [w1515]
      tunnel: w1502 -> [w1514]
      tunnel: [w1566] -> w1504
      tunnel: w1508 -> [w1588]
      tunnel: w1506 -> [w1585]
      tunnel: [w1571] -> w1503
      frame #0 {
        n308 = call "Loop Timer7"("Count(Ticks)"=w1512) -> ("Tick Count(Ticks)"=w1513:u32)
      }
      frame #1 {
        # "(need 4 channels/APD)"
        n309 = xnode "FPGA I/O Node"("Connector0/DIO4"=w1514, "Connector0/DIO5"=w1514, "Connector0/DIO6"=w1514, "Connector0/DIO7"=w1514) -> ()  [unwired: 4 in, 4 out]
      }
      frame #2 {
        n310 = feedback #27(TRUE) -> (w1574:bool)
        n311 = feedback #28(w1588) -> (w1587:u32)
        n312 = Not(x=w1574) -> (.not. x?=w1570:bool)
        n313 = Subtract(x=w1588, y=w1587) -> (x-y=w1586:u32)
        n314 = Select(t="APD Gate ON Count", s=w1570, f="APD Gate OFF Count") -> (s? t:f=w1576:u32)
        n315 = Subtract(x=w1586, y=w1585) -> (x-y=w1577:u32)
        n316 = Subtract(x=w1576, y=w1577) -> (x-y=w1565:u32)
        n317 = Greater?(x=w1577, y=u32 0) -> (0:w1581:bool)
        "APD 1 Gate Late?" <- w1581
        n318 = Boolean To (0,1)(Boolean="+ phase (APD 1 Gate)") -> (0, 1=w1563:i16)
        n319 = Multiply(x=w1563, y="Phase count adjustment (APD 1 Gate)") -> (x*y=w1561:i16)
        n320 = feedback #29(u32 0) -> (w1583:u32)
        n321 = Increment(x=w1583) -> (x+1=w1582:u32)
        n322 = Select(t=w1582, s=w1581, f=w1583) -> (s? t:f=w1580:u32)
        "APD 1 Gate Late Counter" <- w1580
        n323 = Add(x=w1565, y=w1561) -> (x+y=w1566:u32)
        n324 = feedback #30(i16 0) -> (w1568:i16)
        n325 = Subtract(x=w1568, y=w1561) -> (x-y=w1567:i16)
        "APD 1 Gate Relative Phase" <- w1567
        n326 = case shown="2" "APD Gate Operating Mode" {
          tunnel: [TRUE FALSE w1594] -> w1571
          tunnel: w1574 -> [_ _ w1591]
          frame #0 {
          }
          frame #1 {
          }
          frame #2 {
            n327 = Not(x=w1591) -> (.not. x?=w1593:bool)
            n328 = Select(t=w1593, s="Invert APD Gate", f=w1591) -> (s? t:f=w1594:bool)
          }
        }
      }
    }
  }
  n329 = while "RF box board direct communication loop" {
    tunnel: w1 -> [_]
    stop <- FALSE stop-if-true
    n330 = case "Whether to use direct communication method (only use one method at a time)" shown="True" "Direct RF Box \nCommunication" {
      frame #0 {
      }
      frame #1 {
        n331 = case shown="True" "Update Data" {
          frame #0 {
          }
          frame #1 {
            n332 = flat-sequence {
              frame #0 {
                n333 = First Call?() -> (First Call?: T/F=w1598:bool)
                n334 = case shown="True" w1598 {
                  frame #0 {
                  }
                  frame #1 {
                    # "If first time data updated, be sure to set WR high\nbefore setting data and address bits."
                    n335 = flat-sequence {
                      frame #0 {
                        n336 = xnode "FPGA I/O Node"("Connector1/DIO15"=TRUE) -> ()  [unwired: 1 in, 1 out]
                      }
                      frame #1 {
                        n337 = call "Wait"("Count(Ticks)"=u8 40 ("DO Delay 3 (Ticks)")) -> ()  [unwired: 1 out]
                      }
                    }
                  }
                }
              }
              frame #1 {
                n338 = Number To Boolean Array(number="Address") -> (Boolean array=w1660:bool[])
                n339 = Number To Boolean Array(number="Data BD 1") -> (Boolean array=w1661:bool[])
                n340 = Number To Boolean Array(number="Data BD 2") -> (Boolean array=w1630:bool[])
                n341 = Index Array(array=w1661, index=7) -> (element=w1645:bool)
                n342 = Index Array(array=w1661, index=6) -> (element=w1644:bool)
                n343 = Index Array(array=w1661, index=5) -> (element=w1643:bool)
                n344 = Index Array(array=w1661, index=4) -> (element=w1642:bool)
                n345 = Index Array(array=w1661, index=3) -> (element=w1641:bool)
                n346 = Index Array(array=w1661, index=2) -> (element=w1640:bool)
                n347 = Index Array(array=w1661, index=1) -> (element=w1639:bool)
                n348 = Index Array(array=w1661, index=0) -> (element=w1638:bool)
                n349 = Index Array(array=w1660, index=5) -> (element=w1637:bool)
                n350 = Index Array(array=w1660, index=4) -> (element=w1636:bool)
                n351 = Index Array(array=w1660, index=3) -> (element=w1635:bool)
                n352 = Index Array(array=w1660, index=2) -> (element=w1634:bool)
                n353 = Index Array(array=w1660, index=1) -> (element=w1633:bool)
                n354 = Index Array(array=w1660, index=0) -> (element=w1632:bool)
                n355 = Index Array(array=w1630, index=7) -> (element=w1621:bool)
                n356 = Index Array(array=w1630, index=6) -> (element=w1620:bool)
                n357 = Index Array(array=w1630, index=5) -> (element=w1619:bool)
                n358 = Index Array(array=w1630, index=4) -> (element=w1618:bool)
                n359 = Index Array(array=w1630, index=3) -> (element=w1617:bool)
                n360 = Index Array(array=w1630, index=2) -> (element=w1616:bool)
                n361 = Index Array(array=w1630, index=1) -> (element=w1615:bool)
                n362 = Index Array(array=w1630, index=0) -> (element=w1614:bool)
                n363 = xnode "FPGA I/O Node"("Connector1/DIO0"=w1645, "Connector1/DIO1"=w1644, "Connector1/DIO2"=w1643, "Connector1/DIO3"=w1642, "Connector1/DIO4"=w1641, "Connector1/DIO5"=w1640, "Connector1/DIO6"=w1639, "Connector1/DIO7"=w1638, "Connector1/DIO8"=w1637, "Connector1/DIO9"=w1636, "Connector1/DIO10"=w1635, "Connector1/DIO11"=w1634, "Connector1/DIO12"=w1633, "Connector1/DIO13"=w1632, "Connector1/DIO20"=w1621, "Connector1/DIO21"=w1620, "Connector1/DIO22"=w1619, "Connector1/DIO23"=w1618, "Connector1/DIO24"=w1617, "Connector1/DIO25"=w1616, "Connector1/DIO26"=w1615, "Connector1/DIO27"=w1614) -> ()  [unwired: 22 in, 22 out]
              }
              frame #2 {
                # "wait and then apply write signal"
                n364 = call "Wait2"("Count(Ticks)"=u8 40 ("DO Delay 1 (Ticks)")) -> ()  [unwired: 1 out]
              }
              frame #3 {
                # "sending bit low writes data to board buffer"
                n365 = xnode "FPGA I/O Node"("Connector1/DIO15"=FALSE) -> ()  [unwired: 1 in, 1 out]
              }
              frame #4 {
                # "wait then return write signal"
                n366 = call "Wait3"("Count(Ticks)"=u8 40 ("DO Delay 2 (Ticks)")) -> ()  [unwired: 1 out]
              }
              frame #5 {
                # "sending bit high makes ready to\nwrite more data"
                n367 = xnode "FPGA I/O Node"("Connector1/DIO15"=TRUE) -> ()  [unwired: 1 in, 1 out]
              }
            }
          }
        }
      }
    }
  }
  n368 = while "Control APD data integration - stream to host" {
    shift-right: [w1982] -> _
    shift-left: w1 -> [w1987]
    stop <- FALSE stop-if-true
    n369 = flat-sequence {
      tunnel: w1987 -> [w1989]
      tunnel: [w1990] -> w1985
      tunnel: [w1989] -> w1983
      tunnel: [w1998] -> w1986
      tunnel: w1985 -> [w1998]
      tunnel: [w1997] -> w1984
      tunnel: w1983 -> [w1997]
      tunnel: [w1996] -> w1981
      tunnel: [w1995] -> w1980
      tunnel: [w2022] -> w1982
      tunnel: w1986 -> [w2047]
      tunnel: w1984 -> [w2044]
      tunnel: w1981 -> [w2015]
      tunnel: w1980 -> [w2014]
      frame #0 {
        n370 = call "Loop Timer6"("Count(Ticks)"=w1989) -> ("Tick Count(Ticks)"=w1990:u32)
      }
      frame #1 {
        n371 = flat-sequence {
          tunnel: [w1999] -> w1994
          tunnel: w1994 -> [w2002]
          tunnel: [w2004] -> w1993
          tunnel: [w2003] -> w1992
          tunnel: [w2002] -> w1991
          tunnel: [w2010] -> w1995
          tunnel: [w2011] -> w1996
          tunnel: w1993 -> [w2011]
          tunnel: w1992 -> [w2010]
          tunnel: w1991 -> [w2009]
          frame #0 {
            n372 = feedback #31(FALSE) -> (w2000:bool)
            "APD out state" <- w2000
            n373 = Not(x=w2000) -> (.not. x?=w1999:bool)
          }
          frame #1 {
            n374 = local read "APD 1 Counts 1"() -> (w2008:u32)
            n375 = local read "APD 1 Counts 0"() -> (w2007:u32)
            n376 = local read "APD 2 Counts 1"() -> (w2006:u32)
            n377 = local read "APD 2 Counts 0"() -> (w2005:u32)
            n378 = Select(t=w2008, s=w2002, f=w2007) -> (s? t:f=w2004:u32)
            n379 = Select(t=w2006, s=w2002, f=w2005) -> (s? t:f=w2003:u32)
          }
          frame #2 {
            n380 = case shown="False" w2009 {
              frame #0 {
                w2012 = u32 0 ("APD 1 Counts 0")
                n381 = local write "APD 1 Counts 0"(w2012) -> ()
                n382 = local write "APD 2 Counts 0"(w2012) -> ()
              }
              frame #1 {
                w2013 = u32 0 ("APD 1 Counts 1")
                n383 = local write "APD 1 Counts 1"(w2013) -> ()
                n384 = local write "APD 2 Counts 1"(w2013) -> ()
              }
            }
          }
        }
      }
      frame #2 {
        n385 = feedback #32(w2047) -> (w2046:u32)
        n386 = Subtract(x=w2047, y=w2046) -> (x-y=w2045:u32)
        n387 = Subtract(x=w2045, y=w2044) -> (x-y=w2038:u32)
        n388 = case shown="True" "APD to FIFO" {
          tunnel: w2015 -> [_ w2074]
          tunnel: w2014 -> [_ w2072]
          frame #0 {
          }
          frame #1 {
            n389 = flat-sequence {
              tunnel: 0 ("Timeout") -> [w2076]
              tunnel: w2074 -> [w2077]
              tunnel: [w2076] -> w2073
              tunnel: w2073 -> [w2104]
              tunnel: w2072 -> [w2103]
              frame #0 {
                n390 = xnode ("FIFO Write")("Element"=w2077, "Timeout"=w2076) -> ()  [unwired: 1 in, 2 out]
              }
              frame #1 {
                n391 = xnode ("FIFO Write")("Element"=w2103, "Timeout"=w2104) -> ()  [unwired: 1 in, 2 out]
              }
            }
          }
        }
        n392 = Subtract(x="APD Acq Rate Count", y=w2038) -> (x-y=w2023:u32)
        n393 = Greater?(x=w2038, y=u32 0) -> (0:w2040:bool)
        "APD Acq Late?" <- w2040
        n394 = feedback #33(u32 0) -> (w2042:u32)
        n395 = Increment(x=w2042) -> (x+1=w2041:u32)
        n396 = Select(t=w2041, s=w2040, f=w2042) -> (s? t:f=w2039:u32)
        "APD Acq Late Counter" <- w2039
        n397 = Boolean To (0,1)(Boolean="+ phase (APD Acq)") -> (0, 1=w2019:i16)
        n398 = Multiply(x=w2019, y="Phase Count Adjustment (APD Acq)") -> (x*y=w2016:i16)
        n399 = Add(x=w2023, y=w2016) -> (x+y=w2022:u32)
        n400 = feedback #34(i16 0) -> (w2021:i16)
        n401 = Subtract(x=w2021, y=w2016) -> (x-y=w2018:i16)
        "APD Acq Relative Phase" <- w2018
        n402 = To Word Integer(number=w2015) -> (16bit integer=w2031:i16)
        n403 = To Word Integer(number=w2014) -> (16bit integer=w2032:i16)
        n404 = Multiply(x="APD 1 AO scale factor", y=w2031) -> (x*y=w2030:i16)
        n405 = Multiply(x="APD 2 AO scale factor", y=w2032) -> (x*y=w2029:i16)
        n406 = Add(x="APD 1 AO offset", y=w2030) -> (x+y=w2028:i16)
        n407 = Add(x=w2029, y="APD 2 AO offset") -> (x+y=w2026:i16)
        n408 = xnode "FPGA I/O Node"("Connector0/AO6"=w2028, "Connector0/AO7"=w2026) -> ()  [unwired: 2 in, 2 out]
      }
    }
  }
  n409 = timed-loop "RF box board DIO control: control bits" {
    timing: w4 -> [_]
    timing-out: [_] -> w3
    tunnel: [w2130] -> _
    tunnel: w1 -> [w2130]
    stop <- FALSE stop-if-true
    n410 = xnode "FPGA I/O Node"("Connector1/DIO16"="RD", "Connector1/DIO17"="PMODE", "Connector1/DIO18"="OSK Bd 1", "Connector1/DIO19"="Reset Bd 1", "Connector1/DIO28"="OSK Bd 2", "Connector1/DIO29"="Reset Bd 2") -> ()  [unwired: 6 in, 6 out]
  }
  n411 = while "Green fluorescent laser interlacing (DO to IA 532 nm AOM ME amp)." {
    shift-right: [w2221] -> _
    shift-left: w1 -> [w2226]
    shift-right: [w2220] -> _
    shift-left: FALSE -> [w2218]
    stop <- FALSE stop-if-true
    n412 = flat-sequence {
      tunnel: w2226 -> [w2229]
      tunnel: [w2230] -> w2224
      tunnel: [w2229] -> w2222
      tunnel: [w2228] -> w2219
      tunnel: w2218 -> [w2228]
      tunnel: [w2233] -> w2225
      tunnel: w2224 -> [w2233]
      tunnel: [w2232] -> w2223
      tunnel: w2222 -> [w2232]
      tunnel: w2219 -> [w2231]
      tunnel: [w2273] -> w2221
      tunnel: w2225 -> [w2300]
      tunnel: w2223 -> [w2297]
      tunnel: [w2283] -> w2220
      frame #0 {
        n413 = call "Loop Timer4"("Count(Ticks)"=w2229) -> ("Tick Count(Ticks)"=w2230:u32)
      }
      frame #1 {
        n414 = xnode "FPGA I/O Node"("Connector1/DIO37"=w2231, "Connector1/DIO38"=w2231, "Connector1/DIO39"=w2231) -> ()  [unwired: 3 in, 3 out]
      }
      frame #2 {
        n415 = feedback #35(w2300) -> (w2299:u32)
        n416 = Subtract(x=w2300, y=w2299) -> (x-y=w2298:u32)
        n417 = Subtract(x=w2298, y=w2297) -> (x-y=w2289:u32)
        n418 = Greater?(x=w2289, y=u32 0) -> (0:w2293:bool)
        "GI Late?" <- w2293
        n419 = Boolean To (0,1)(Boolean="+ phase (GI)") -> (0, 1=w2278:i16)
        n420 = Multiply(x=w2278, y="Phase count adjustment (GI)") -> (x*y=w2275:i16)
        n421 = feedback #36(u32 0) -> (w2295:u32)
        n422 = Increment(x=w2295) -> (x+1=w2294:u32)
        n423 = Select(t=w2294, s=w2293, f=w2295) -> (s? t:f=w2292:u32)
        "GI Late Counter" <- w2292
        n424 = feedback #37(i16 0) -> (w2276:i16)
        n425 = Subtract(x=w2276, y=w2275) -> (x-y=w2274:i16)
        "GI Relative phase" <- w2274
        n426 = feedback #38(TRUE) -> (w2286:bool)
        n427 = case shown="2" "Operating Mode" {
          tunnel: [TRUE FALSE w2306] -> w2283
          tunnel: w2286 -> [_ _ w2303]
          frame #0 {
          }
          frame #1 {
          }
          frame #2 {
            n428 = Not(x=w2303) -> (.not. x?=w2305:bool)
            n429 = Select(t=w2305, s="Invert GI", f=w2303) -> (s? t:f=w2306:bool)
          }
        }
        n430 = Not(x=w2286) -> (.not. x?=w2282:bool)
        n431 = Select(t="Green interlace ON count", s=w2282, f="Green interlace OFF count") -> (s? t:f=w2288:u32)
        n432 = Subtract(x=w2288, y=w2289) -> (x-y=w2279:u32)
        n433 = Add(x=w2279, y=w2275) -> (x+y=w2273:u32)
      }
    }
  }
  n434 = while "Green fluorescent laser interlacing (Current to IA 532 nm AOM ME amp)." {
    shift-right: [w2312] -> _
    shift-left: w1 -> [w2315]
    shift-right: [w2309] -> _
    shift-left: w1 -> [w2307]
    stop <- FALSE stop-if-true
    n435 = flat-sequence {
      tunnel: w2315 -> [w2318]
      tunnel: [w2319] -> w2314
      tunnel: [w2318] -> w2313
      tunnel: [w2317] -> w2308
      tunnel: w2307 -> [w2317]
      tunnel: [w2322] -> w2311
      tunnel: w2314 -> [w2322]
      tunnel: [w2321] -> w2310
      tunnel: w2313 -> [w2321]
      tunnel: w2308 -> [w2320]
      tunnel: [w2335] -> w2312
      tunnel: [w2353] -> w2309
      tunnel: w2311 -> [w2372]
      tunnel: w2310 -> [w2369]
      frame #0 {
        n436 = call "Loop Timer10"("Count(Ticks)"=w2318) -> ("Tick Count(Ticks)"=w2319:u32)
      }
      frame #1 {
        n437 = xnode "FPGA I/O Node"("Chassis2/Mod4/AO0"=w2320) -> ()  [unwired: 1 in, 1 out]
      }
      frame #2 {
        n438 = Subtract(x="Green interlace OFF count 2", y="Green int current ON count adj") -> (x-y=w2345:u32)
        n439 = feedback #39(w2372) -> (w2371:u32)
        n440 = Add(x="Green int current ON count adj", y="Green interlace ON count 2") -> (x+y=w2346:u32)
        n441 = Subtract(x=w2372, y=w2371) -> (x-y=w2370:u32)
        n442 = Subtract(x=w2370, y=w2369) -> (x-y=w2361:u32)
        n443 = Greater?(x=w2361, y=u32 0) -> (0:w2365:bool)
        "GI Late? 2" <- w2365
        n444 = Boolean To (0,1)(Boolean="+ phase (GI) 2") -> (0, 1=w2341:i16)
        n445 = Multiply(x=w2341, y="Phase count adjustment (GI) 2") -> (x*y=w2337:i16)
        n446 = feedback #40(u32 0) -> (w2367:u32)
        n447 = Increment(x=w2367) -> (x+1=w2366:u32)
        n448 = Select(t=w2366, s=w2365, f=w2367) -> (s? t:f=w2364:u32)
        "GI Late Counter 2" <- w2364
        n449 = feedback #41(i16 0) -> (w2338:i16)
        n450 = Subtract(x=w2338, y=w2337) -> (x-y=w2336:i16)
        "GI Relative phase 2" <- w2336
        n451 = feedback #42(TRUE) -> (w2358:bool)
        n452 = case shown="2" "Operating Mode 2" {
          tunnel: [TRUE FALSE w2389] -> w2347
          tunnel: w2358 -> [_ _ w2386]
          frame #0 {
          }
          frame #1 {
          }
          frame #2 {
            n453 = Not(x=w2386) -> (.not. x?=w2388:bool)
            n454 = Select(t=w2388, s="Invert GI 2", f=w2386) -> (s? t:f=w2389:bool)
          }
        }
        n455 = And(x=w2347, y="Green FB On/Off") -> (x .and. y?=w2348:bool)
        n456 = case shown="True" w2348 {
          tunnel: "Current Out" -> [w2373 _]
          tunnel: [w2373 w2378] -> w2352
          frame #0 {
          }
          frame #1 {
            n457 = local read "Green FB Sum"() -> (w2374:i16)
            n458 = call "Slower PID.vi"("process variable"=w2374, "reset?"="Green FB Reset", "setpoint"="Green FB Setpoint", "PID gains (x 2^8)"="Green FB Gains", "output range"=cluster{"output high":i16, "output low":i16} {"output high"=32767, "output low"=-32768} ("Green FB output range")) -> ("output"=w2382:i16)  [unwired: 10 out]
            n459 = To Long Integer(number=w2382) -> (32bit integer=w2375:i32)
            n460 = Add(x=w2375, y=32768) -> (x+y=w2377:i32)
            n461 = To Unsigned Word Integer(number=w2377) -> (unsigned 16bit integer=w2378:u16)
          }
        }
        n462 = Not(x=w2358) -> (.not. x?=w2355:bool)
        n463 = Select(t=w2346, s=w2355, f=w2345) -> (s? t:f=w2360:u32)
        n464 = Subtract(x=w2360, y=w2361) -> (x-y=w2339:u32)
        n465 = Add(x=w2339, y=w2337) -> (x+y=w2335:u32)
        n466 = Boolean To (0,1)(Boolean=w2347) -> (0, 1=w2354:i16)
        n467 = To Unsigned Word Integer(number=w2354) -> (unsigned 16bit integer=w2351:u16)
        n468 = Multiply(x=w2351, y=w2352) -> (x*y=w2353:u16)
      }
    }
  }
  n469 = while "Green excitation laser feedback measurement" {
    shift-right: [w2390] -> _
    shift-left: w1 -> [w2395]
    stop <- FALSE stop-if-true
    n470 = flat-sequence {
      tunnel: w2395 -> [w2397]
      tunnel: [w2398] -> w2393
      tunnel: [w2397] -> w2391
      tunnel: [w2405] -> w2394
      tunnel: w2393 -> [w2405]
      tunnel: [w2404] -> w2392
      tunnel: w2391 -> [w2404]
      tunnel: [w2481] -> w2390
      tunnel: w2394 -> [w2499]
      tunnel: w2392 -> [w2496]
      frame #0 {
        n471 = call "Loop Timer9"("Count(Ticks)"=w2397) -> ("Tick Count(Ticks)"=w2398:u32)
      }
      frame #1 {
        n472 = xnode "FPGA I/O Node"("Connector1/DIO35"=TRUE) -> ("Chassis2/Mod1/AI0"=w2403:i16, "Chassis2/Mod1/AI1"=w2402:i16, "Chassis2/Mod1/AI2"=w2399:i16)  [unwired: 4 in, 4 out]
        "Green FB Sum" <- w2399
        n473 = Bundle("Chassis2/Mod1/AI0"=w2403, "Chassis2/Mod1/AI1"=w2402, "Chassis2/Mod1/AI2"=w2399) -> (→"Green FB Signals":T12)  [unwired: 1 out]
      }
      frame #2 {
        n474 = feedback #43(w2499) -> (w2498:u32)
        n475 = Subtract(x=w2499, y=w2498) -> (x-y=w2497:u32)
        n476 = xnode "FPGA I/O Node"("Connector1/DIO35"=FALSE) -> ()  [unwired: 1 in, 1 out]
        n477 = Subtract(x=w2497, y=w2496) -> (x-y=w2490:u32)
        n478 = Subtract(x="Green FB Count", y=w2490) -> (x-y=w2485:u32)
        n479 = Greater?(x=w2490, y=u32 0) -> (0:w2492:bool)
        "Green FB Late?" <- w2492
        n480 = Boolean To (0,1)(Boolean="+ phase (Green FB)") -> (0, 1=w2483:i16)
        n481 = Multiply(x=w2483, y="Phase count adjustment (Green FB)") -> (x*y=w2478:i16)
        n482 = feedback #44(u32 0) -> (w2494:u32)
        n483 = Increment(x=w2494) -> (x+1=w2493:u32)
        n484 = Select(t=w2493, s=w2492, f=w2494) -> (s? t:f=w2491:u32)
        "Green Late Counter" <- w2491
        n485 = Add(x=w2485, y=w2478) -> (x+y=w2481:u32)
        n486 = feedback #45(i16 0) -> (w2480:i16)
        n487 = Subtract(x=w2480, y=w2478) -> (x-y=w2479:i16)
        "Green FB Relative Phase" <- w2479
      }
    }
  }
  n488 = while "Control Additional IO (Green laser flip mount)" {
    stop <- FALSE stop-if-true
    n489 = xnode "FPGA I/O Node"("Connector0/DIO3"="Green Filter Flipper", "Connector0/DIO2"="Connector0/DIO9", "Connector1/DIO32"="Connector1/DIO32", "Connector1/DIO33"="Connector1/DIO33", "Connector1/DIO34"="Connector1/DIO34", "Chassis2/Mod4/AO1"="Chassis2/Mod4/AO1") -> ()  [unwired: 6 in, 6 out]
    n490 = call "Loop Timer2"("Count(Ticks)"="Extra DO Counts") -> ()  [unwired: 1 out]
  }
  n491 = node-c288(w3) -> ()
